vi "KickToPassReceiverTactic.vi"(7 "first call":bool, 8 "error in (no error)":errorcluster, 9 "Robot":refnum<class "Robot.lvclass">, 10 "Game in":refnum<class "Game.lvclass">, 11 "KickToPassReceiverTactic in":refnum<class "KickToPassReceiverTactic.lvclass">) -> (0 "error out":errorcluster, 2 "Robot out":refnum<class "Robot.lvclass">, 3 "KickToPassReceiverTactic out":refnum<class "KickToPassReceiverTactic.lvclass">)   [LabVIEW 2020, in "KickToPassReceiverTactic.lvclass"]
uses:
  KickToPassReceiverTactic.lvclass
  Robot_class/Robot.lvclass
  Game_class/Game.lvclass
  Robot_class/Robot.lvclass/Robot.ctl
  Robot_class/tactics.ctl
  Team_class/OffensivePlay.ctl
  KickToPassReceiverTacticStates.ctl
  Tactic_class/Tactic.lvclass/Tactic.ctl
  Game_class/Game.lvclass/Game.ctl
  Parameters_class/Parameters.lvclass/Parameters.ctl
  Team_class/Team.lvclass/Team.ctl
  Robot_class/roles.ctl
  Object_class/Object.lvclass/Object.ctl
  Skillbook_class/Skillbook.lvclass/Skillbook.ctl
  Events_class/Events.lvclass/Events.ctl
  KickToPassReceiverTactic.lvclass/KickToPassReceiverTactic.ctl
  Robot_class/Read role.vi
  Object_class/Read x.vi
  Object_class/Read y.vi
  Events_class/Read kick.vi
  Events_class/Read touch.vi
  Game_class/Read EventsRef.vi
  Game_class/Read OffensiveTeam.vi
  Team_class/Read OffensivePlay.vi
  Skillbook_class/Read KickToSkill.vi
  Skillbook_class/Read HaltSkill.vi
  Skillbook_class/Read TableReceiverGoToSkill.vi
  Game_class/Read Parameters.lvclass.vi
  Game_class/Read Utilities.lvclass.vi
  Game_class/Read BallRef.vi
  Game_class/Read FieldRef.vi
  Team_class/Read RobotRef.vi
  Parameters_class/Read AttakingOurselves.vi
  Tactic_class/Read Skillbook.vi
  Write States.vi
  Robot_class/Write tactic.vi
  Ally_class/Ally.lvclass
  Ball_class/Ball.lvclass
  Parameters_class/Parameters.lvclass
  Utilities_class/Utilities.lvclass
  Field_class/Field.lvclass
  Skillbook_class/Skillbook.lvclass
  Events_class/Events.lvclass
  KickToSkill_class/KickToSkill.lvclass
  HaltSkill_class/HaltSkill.lvclass
  TableReceiverGoToSkill_class/TableReceiverGoToSkill.lvclass
panel:
  out "x .or. y?":bool
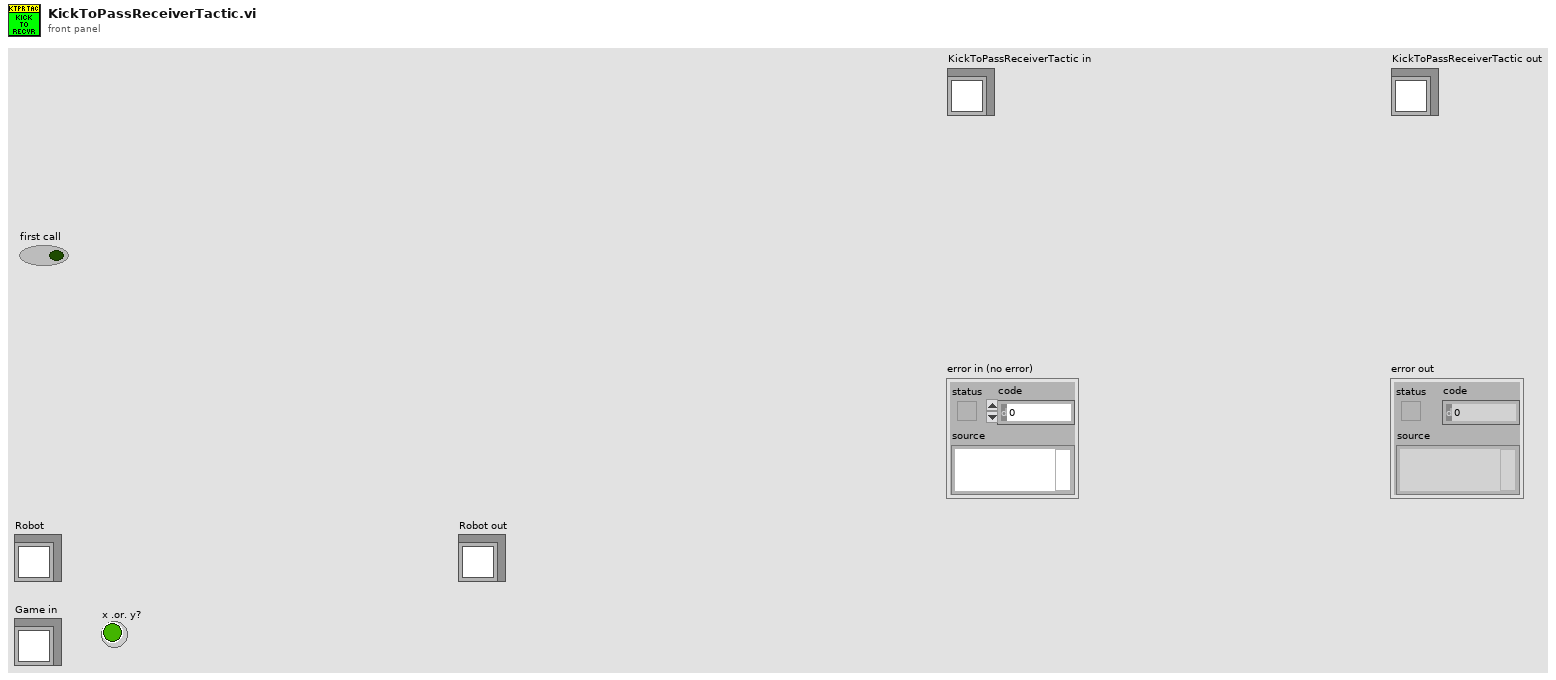
[diagram p1: front panel]
types:
  T1 = typedef "KickToPassReceiverTacticStates.ctl" = enum16{"Halt", "GoToReceiveTable", "KickToPassReceiver", "WaitPass", "Exit"}
  T2 = typedef "OffensivePlay.ctl" = enum16{"KeeperPassToStriker", "PrepareKeeperPass", "ACBPass", "ABCPass", "PrepareTriplePass", "TableWithStriker", "TableWith2ndStrikerPlay", "PrepareDoublePass", "PrepareRollToPass", "SimplePass", "PreparePass", "PassToStriker", "BallOutOfField", "PassTo2ndStriker", "StopOffensive", "Prepare Penalty Enemy", "EnemyPossessionAtEnemyField", "EnemyPossesionAtOurField", "TestPlay", "PreparePenaltyAlly", "KickPenaltyAlly", "PrepareKickoffAlly", "PrepareKickoffEnemy", "IndirectEnemy", "DirectEnemy", "PreparePassInGame1", "NormalGame", "DirectKick", "Pass", "Halt", "Timeout", "PassPlay", "PenaltyEnemy"}
  T3 = typedef "tactics.ctl" = enum16{"ReceivePassInFuturePoint", "Roller", "PrepareRollToPassRollerGoTo", "PrepareRollToPassReceiverGoTo", "WaitRoll", "PositionToRoll", "PenaltyAttacker", "PassObserver", "PenaltyDefense", "TableReceiverTactic", "Test", "DefendGoal", "Marker", "FollowAttacker", "DefendArea", "Shoot", "AttackerAimGoal", "AttackerBallOutOfField", "AttackerBlock", "AttackerStop", "Duelist", "Halt", "ZigZag", "GoTo", "Timeout", "KickToPassReceiver", "PositionToReceivePass", "WaitPass"}
  T4 = typedef "roles.ctl" = enum16{"SecondMarker", "WaitPass", "ABCThirdKicker", "ABCFirstKicker", "ABCSecondKicker", "Tabler", "TableFinalizer", "PrepareRollToPassRoller", "PrepareRollToPassReceiver", "SimplePassRoll", "SimplePassRollReceiver", "PenaltyDefense", "PreparePassReceiver 2", "PreparePassReceiver 1", "PassObserver", "Timeout", "Goto", "ZigZag", "None", "BallOutOfField", "DefenderArea", "Duelist", "AttackerStop", "FollowAttacker", "KeeperRole", "KickPenalty", "AttackerAimGoal", "AttackerBlock", "Marker", "Halt", "Shoot", "PassKicker", "PassReceiver", "TestRole", "PenaltyAttacker"}
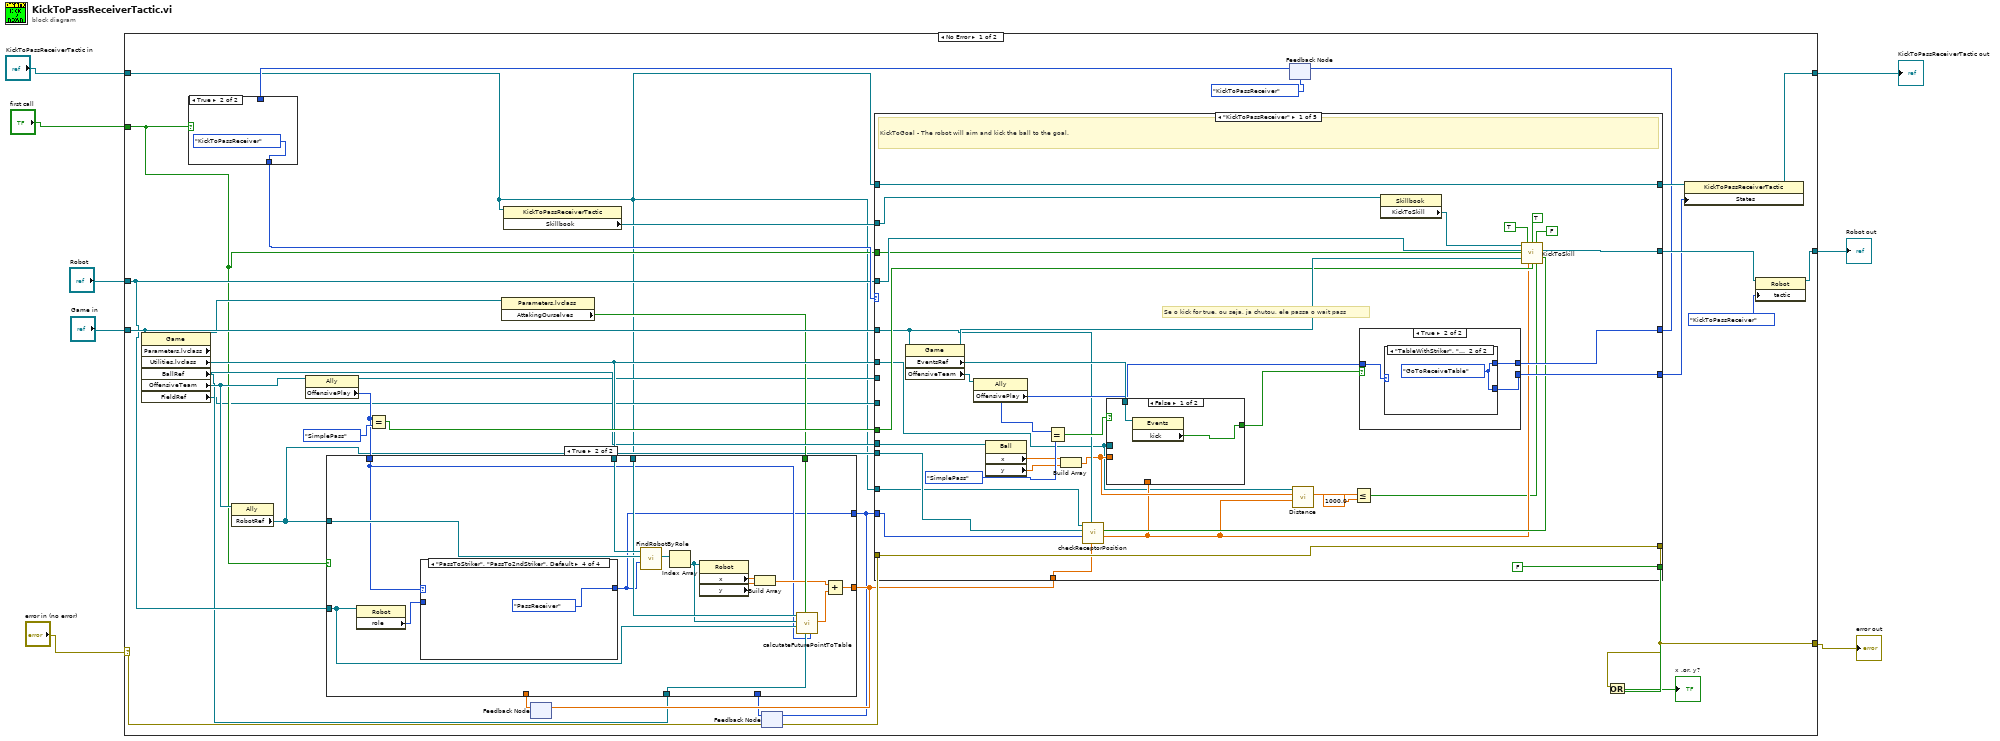
[diagram p0: block diagram]
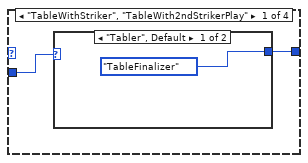
[diagram p3: hidden frame]
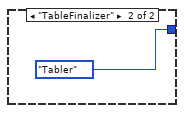
[diagram p4: hidden frame]
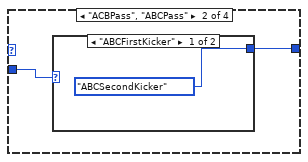
[diagram p5: hidden frame]
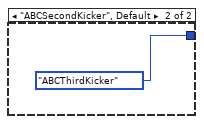
[diagram p6: hidden frame]
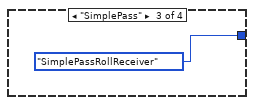
[diagram p7: hidden frame]
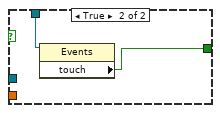
[diagram p9: hidden frame]
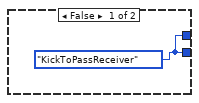
[diagram p10: hidden frame]
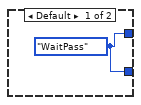
[diagram p11: hidden frame]
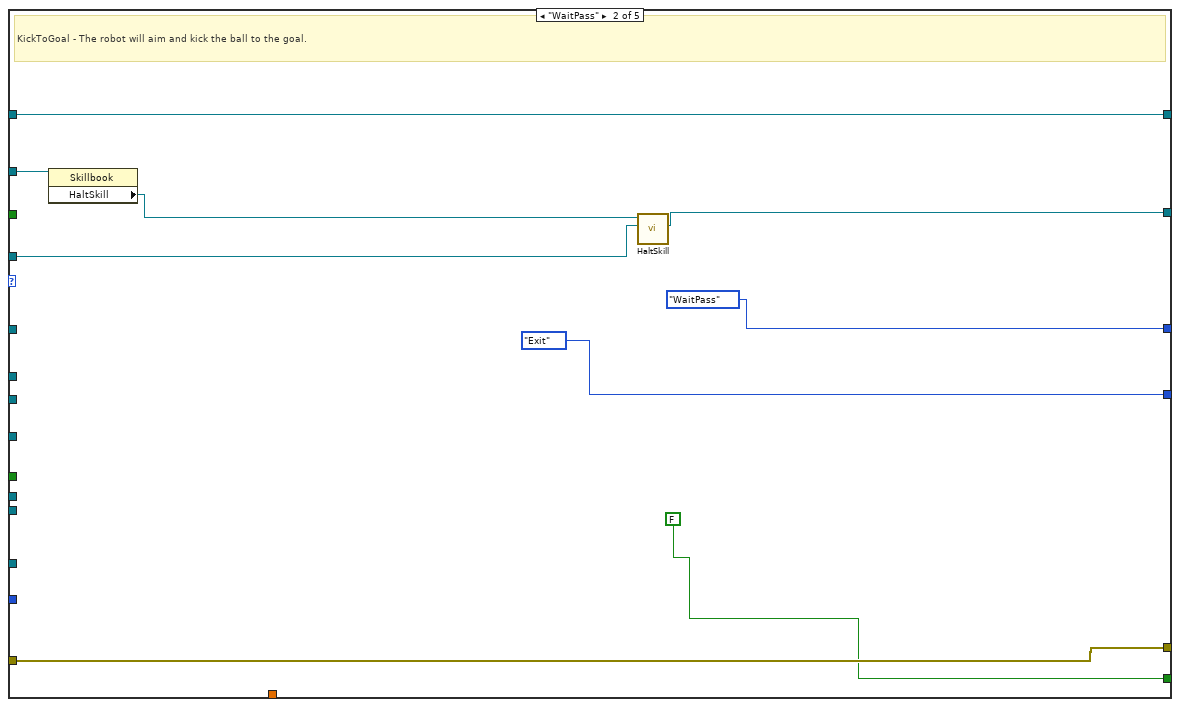
[diagram p12: hidden frame]
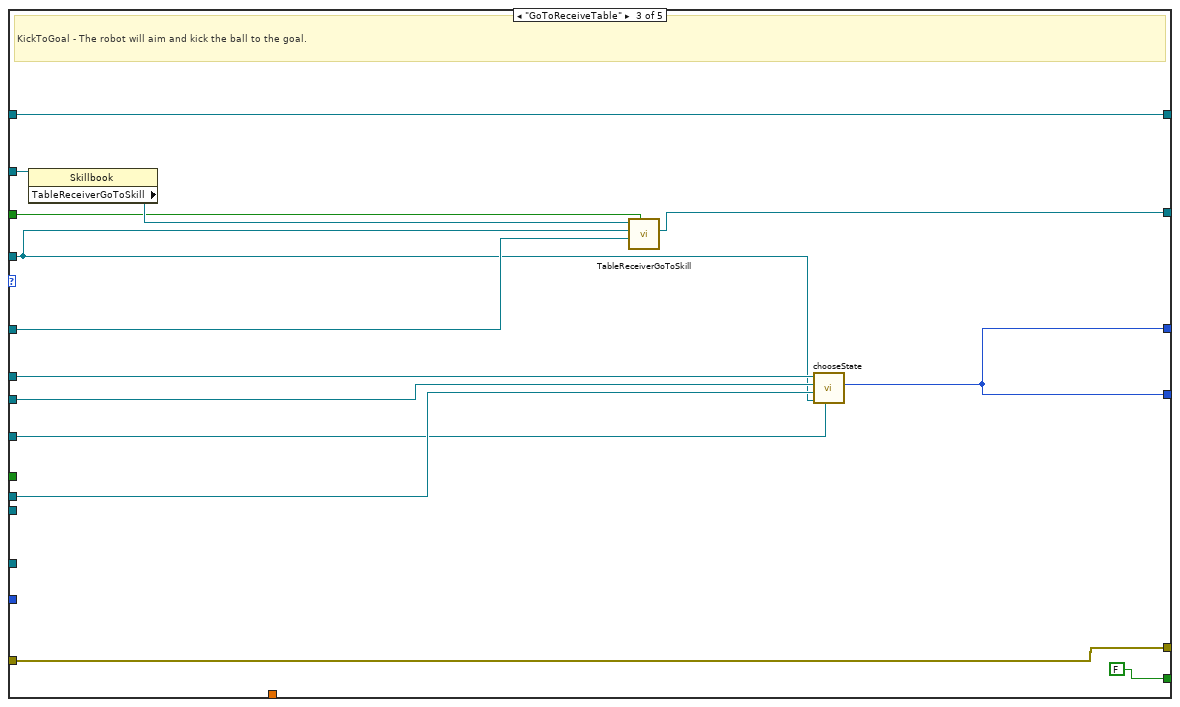
[diagram p13: hidden frame]
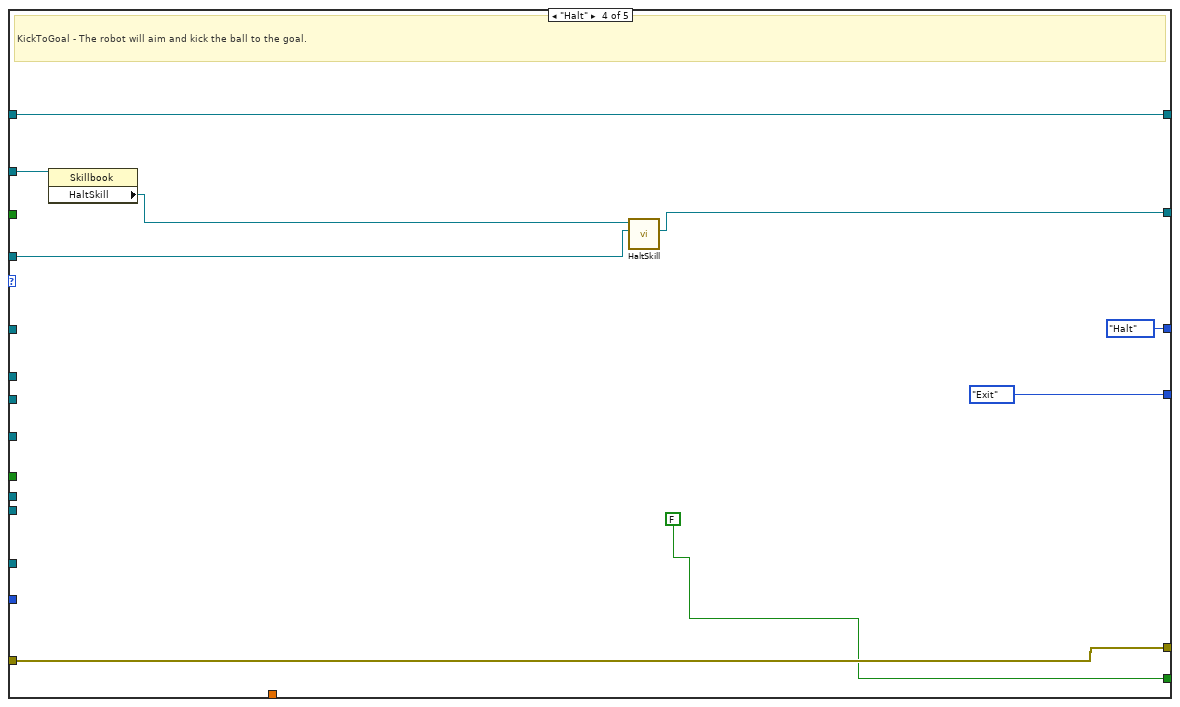
[diagram p14: hidden frame]
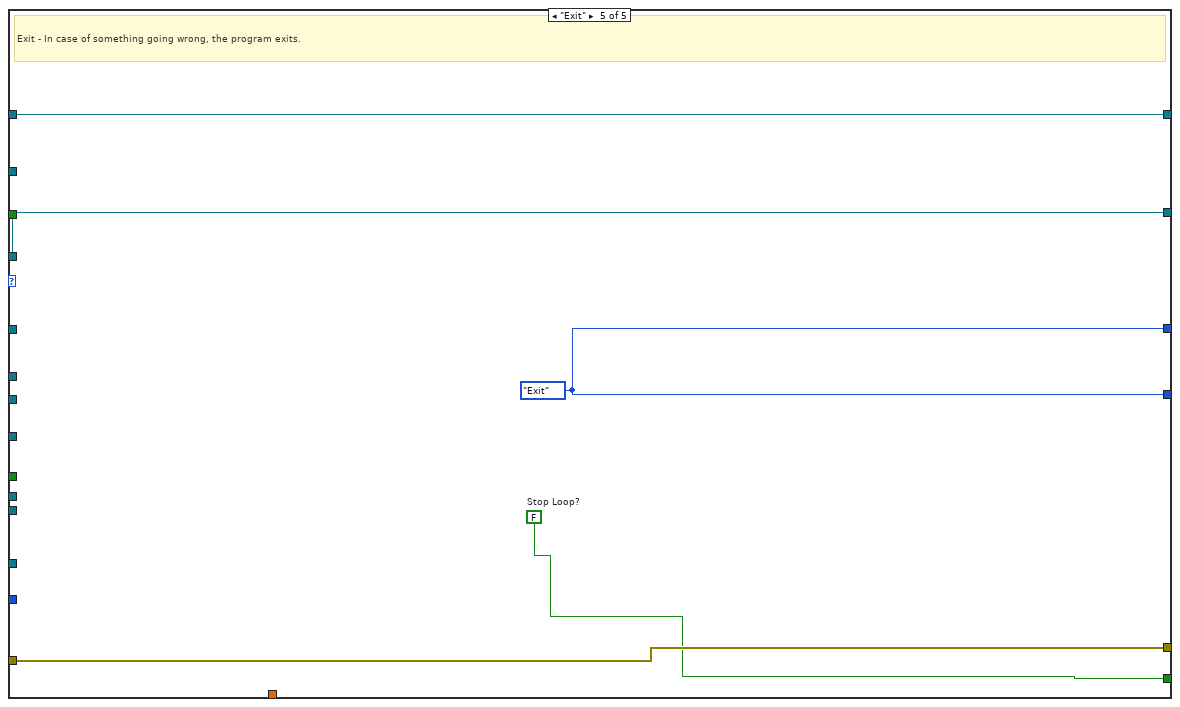
[diagram p15: hidden frame]
diagram:
  n1 = case shown="No Error" "error in (no error)" {
    selector: "error in (no error)" -> [w36 w158]
    tunnel: [w37 w158] -> w2
    tunnel: [w38 w157] -> w3
    tunnel: "KickToPassReceiverTactic in" -> [w9 w157]
    tunnel: "Robot" -> [w23 w156]
    tunnel: "Game in" -> [w35 _]
    tunnel: [w30 w156] -> w6
    tunnel: "first call" -> [w14 _]
    frame No Error {
      n2 = property class="Game"(reference=w35) -> ("Parameters.lvclass"=w20:refnum<class "Parameters.lvclass">, "Utilities.lvclass"=w25:refnum<class "Utilities.lvclass">, "BallRef"=w21:refnum<class "Ball.lvclass">, "OffensiveTeam"=w28:refnum<class "Ally.lvclass">, "FieldRef"=w13:refnum<class "Field.lvclass">)  [unwired: 1 in, 2 out]
      n3 = property class="Ally"(reference=w28) -> ("RobotRef"=w10:refnum<class "Robot.lvclass">[])  [unwired: 1 in, 2 out]
      n4 = property class="Ally"(reference=w28) -> (reference out=w15:refnum<class "Ally.lvclass">, "OffensivePlay"=w24:T2)  [unwired: 1 in, 1 out]
      n5 = Equal?(x=w24, y=OffensivePlay."SimplePass" ("OffensivePlay")) -> (x = y?=w27:bool)
      n6 = property class="Parameters.lvclass"(reference=w20) -> ("AttakingOurselves"=w19:bool)  [unwired: 1 in, 2 out]
      n7 = property class="KickToPassReceiverTactic"(reference=w9) -> ("Skillbook"=w40:refnum<class "Skillbook.lvclass">)  [unwired: 1 in, 2 out]
      n8 = feedback #1() -> (w26:dbl[])  [unwired: 1 in]
      n9 = feedback #2() -> (w11:T4)  [unwired: 1 in]
      n10 = case shown="True" w14 {
        tunnel: w10 -> [_ w60]
        tunnel: w26 -> [w44 _]
        tunnel: w25 -> [_ w59]
        tunnel: w24 -> [_ w46]
        tunnel: w23 -> [_ w48]
        tunnel: [w44 w55] -> w22
        tunnel: w21 -> [_ w47]
        tunnel: w19 -> [_ w52]
        tunnel: w9 -> [_ w51]
        tunnel: [w43 w45] -> w12
        tunnel: w11 -> [w43 _]
        frame False {
        }
        frame True {
          n11 = property class="Robot"(reference=w48) -> ("role"=w54:T4)  [unwired: 1 in, 2 out]
          n12 = case shown="\"PassToStriker\", \"PassTo2ndStriker\", Default" w46 {
            tunnel: [w62 w65 roles."SimplePassRollReceiver" ("role") roles."PassReceiver" ("role")] -> w45
            tunnel: w54 -> [w61 w66 _ _]
            frame "TableWithStriker", "TableWith2ndStrikerPlay" {
              n13 = case shown="\"Tabler\", Default" w61 {
                tunnel: [roles."TableFinalizer" ("role") roles."Tabler" ("role")] -> w62
                frame "Tabler", Default {
                }
                frame "TableFinalizer" {
                }
              }
            }
            frame "ACBPass", "ABCPass" {
              n14 = case shown="\"ABCFirstKicker\"" w66 {
                tunnel: [roles."ABCSecondKicker" ("role") roles."ABCThirdKicker" ("role")] -> w65
                frame "ABCFirstKicker" {
                }
                frame "ABCSecondKicker", Default {
                }
              }
            }
            frame "SimplePass" {
            }
            frame "PassToStriker", "PassTo2ndStriker", Default {
            }
          }
          n15 = call "FindRobotByRole.vi"("role"=w45, "RobotRef"=w60, "Utilities in"=w59) -> ("Robots"=w58:refnum<class "Robot.lvclass">[])  [unwired: 6 in, 2 out]
          n16 = Index Array(array=w58) -> (element=w49:refnum<class "Robot.lvclass">)  [unwired: 1 in]
          n17 = property class="Robot"(reference=w49) -> ("x"=w57:dbl, "y"=w56:dbl)  [unwired: 1 in, 2 out]
          n18 = Build Array(w57, w56) -> (w50:dbl[])
          n19 = call "calcutateFuturePointToTable.vi"("OffensivePlay"=w46, "BallRef"=w47, "AttackingOurselves?"=w52, "Robot that\nmake the pass"=w48, "Robot that will\nreceive the pass"=w49, "KickToPassReceiverTactic in"=w51) -> ("Array to Receiver trajectory"=w53:dbl[])  [unwired: 3 in, 2 out]
          n20 = Add(x=w50, y=w53) -> (x+y=w55:dbl[])
        }
      }
      n21 = feedback-in #1(w22) -> ()
      n22 = feedback-in #2(w12) -> ()
      n23 = feedback #3(KickToPassReceiverTacticStates."KickToPassReceiver" ("States")) -> (w33:T1)
      n24 = case shown="True" w14 {
        tunnel: [w71 KickToPassReceiverTacticStates."KickToPassReceiver" ("States")] -> w34
        tunnel: w33 -> [w71 _]
        frame False {
        }
        frame True {
        }
      }
      n25 = case shown="\"KickToPassReceiver\"" w34 {
        tunnel: [FALSE ("Stop Loop?") FALSE ("Stop Loop?") FALSE ("Stop Loop?") FALSE ("Stop Loop?") w152] -> w42
        tunnel: w36 -> [w107 w125 w137 w145 w155]
        tunnel: [w107 w125 w137 w145 w155] -> w37
        tunnel: w40 -> [w106 w127 w141 w149 _]
        tunnel: w23 -> [w102 w119 w129 w150 w153]
        tunnel: [w104 w121 w139 w147 w153] -> w31
        tunnel: [w105 w126 w138 w146 w154] -> w39
        tunnel: w9 -> [w105 w126 w138 w146 w154]
        tunnel: w35 -> [w80 _ w131 _ _]
        tunnel: [w100 KickToPassReceiverTacticStates."Exit" ("States") w135 KickToPassReceiverTacticStates."Exit" ("States") w151] -> w16
        tunnel: [w99 KickToPassReceiverTacticStates."WaitPass" ("States") w135 KickToPassReceiverTacticStates."Halt" ("States") w151] -> w17
        tunnel: w21 -> [w91 _ w133 _ _]
        tunnel: w25 -> [w76 _ w134 _ _]
        tunnel: w27 -> [w88 _ _ _ _]
        tunnel: w22 -> [w85 _ _ _ _]
        tunnel: w15 -> [_ _ w132 _ _]
        tunnel: w14 -> [w86 _ w130 _ _]
        tunnel: w13 -> [_ _ w128 _ _]
        tunnel: w12 -> [w81 _ _ _ _]
        tunnel: w10 -> [w83 _ _ _ _]
        tunnel: w9 -> [w82 _ _ _ _]
        frame "KickToPassReceiver" {
          # "Se o kick for true, ou seja, ja chutou, ele passa o wait pass"
          # "KickToGoal - The robot will aim and kick the ball to the goal."
          n26 = property class="Game"(reference=w80) -> (reference out=w101:refnum<class "Game.lvclass">, "EventsRef"=w95:refnum<class "Events.lvclass">, "OffensiveTeam"=w93:refnum<class "Ally.lvclass">)  [unwired: 1 in, 1 out]
          n27 = property class="Ally"(reference=w93) -> ("OffensivePlay"=w87:T2)  [unwired: 1 in, 2 out]
          n28 = property class="Ball"(reference=w91) -> ("x"=w90:dbl, "y"=w89:dbl)  [unwired: 1 in, 2 out]
          n29 = Equal?(x=w87, y=OffensivePlay."SimplePass" ("OffensivePlay")) -> (x = y?=w96:bool)
          n30 = Build Array(w90, w89) -> (w78:dbl[])
          n31 = call "checkReceptorPosition.vi"("target"=w85, "Game"=w80, "role"=w81, "OffensiveRobots"=w83, "KickToPassReceiverTactic in"=w82) -> ("finalTarget"=w77:dbl[], "calculateForce"=w84:bool)  [unwired: 3 in, 2 out]
          n32 = case shown="False" w96 {
            tunnel: w95 -> [w110 w112]
            tunnel: [w109 w111] -> w94
            tunnel: w77 -> [_ _]
            tunnel: w78 -> [_ _]
            tunnel: w76 -> [_ _]
            frame False {
              n33 = property class="Events"(reference=w110) -> ("kick"=w109:bool)  [unwired: 1 in, 2 out]
            }
            frame True {
              n34 = property class="Events"(reference=w112) -> ("touch"=w111:bool)  [unwired: 1 in, 2 out]
            }
          }
          n35 = call-dynamic "Distance.vi"("P1"=w77, "P2"=w78, "Utilities in"=w76) -> ("Distance"=w75:dbl)  [unwired: 6 in, 2 out]
          n36 = Less Or Equal?(x=w75, y=1000.0) -> (x <= y?=w73:bool)
          n37 = case shown="True" w94 {
            tunnel: [w113 w116] -> w100
            tunnel: [w113 w115] -> w99
            tunnel: w87 -> [_ w114]
            frame False {
              w113 = KickToPassReceiverTacticStates."KickToPassReceiver" ("States")
            }
            frame True {
              n38 = case shown="\"TableWithStriker\", \"TableWith2ndStrikerPlay\"" w114 {
                tunnel: [w117 w118] -> w116
                tunnel: [w117 w118] -> w115
                frame Default {
                  w117 = KickToPassReceiverTacticStates."WaitPass" ("States")
                }
                frame "TableWithStriker", "TableWith2ndStrikerPlay" {
                  w118 = KickToPassReceiverTacticStates."GoToReceiveTable" ("States")
                }
              }
            }
          }
          n39 = property class="Skillbook"(reference=w106) -> ("KickToSkill"=w103:refnum<class "KickToSkill.lvclass">)  [unwired: 1 in, 2 out]
          n40 = call "KickToSkill.vi"("KickToSkill in"=w103, "use criteria?"=TRUE, "chipKick ?"=TRUE, "fixTarget"=FALSE, "Robot"=w102, "firstCall?"=w86, "Game"=w101, "calculate force?"=w84, "Target"=w77, "KickForce 0?"=w88, "ForceInGame"=w73) -> ("Robot out"=w104:refnum<class "Robot.lvclass">)  [unwired: 2 in, 2 out]
        }
        frame "WaitPass" {
          # "KickToGoal - The robot will aim and kick the ball to the goal."
          n41 = property class="Skillbook"(reference=w127) -> ("HaltSkill"=w120:refnum<class "HaltSkill.lvclass">)  [unwired: 1 in, 2 out]
          n42 = call-dynamic "HaltSkill.vi"("Robot"=w119, "HaltSkill in"=w120) -> ("Robot out"=w121:refnum<class "Robot.lvclass">)  [unwired: 7 in, 2 out]
        }
        frame "GoToReceiveTable" {
          # "KickToGoal - The robot will aim and kick the ball to the goal."
          n43 = property class="Skillbook"(reference=w141) -> ("TableReceiverGoToSkill"=w140:refnum<class "TableReceiverGoToSkill.lvclass">)  [unwired: 1 in, 2 out]
          n44 = call "TableReceiverGoToSkill.vi"("Firstcall?"=w130, "Game"=w131, "Robot in"=w129, "TableReceiverGoToSkill in"=w140) -> ("Robot out"=w139:refnum<class "Robot.lvclass">)  [unwired: 5 in, 2 out]
          n45 = call "chooseState.vi"("FieldRef"=w128, "Robot"=w129, "BallRef"=w133, "OffensiveTeam"=w132, "Utilities in"=w134) -> ("state"=w135:T1)  [unwired: 6 in]
        }
        frame "Halt" {
          # "KickToGoal - The robot will aim and kick the ball to the goal."
          n46 = property class="Skillbook"(reference=w149) -> ("HaltSkill"=w148:refnum<class "HaltSkill.lvclass">)  [unwired: 1 in, 2 out]
          n47 = call-dynamic "HaltSkill.vi"("Robot"=w150, "HaltSkill in"=w148) -> ("Robot out"=w147:refnum<class "Robot.lvclass">)  [unwired: 7 in, 2 out]
        }
        frame "Exit" {
          w151 = KickToPassReceiverTacticStates."Exit" ("States")
          w152 = FALSE  # Stop Loop?
          # "Exit - In case of something going wrong, the program exits."
        }
      }
      n48 = feedback-in #3(w17) -> ()
      n49 = Or(x=w37, y=w42) -> (x .or. y?=→"x .or. y?":bool)
      n50 = property class="KickToPassReceiverTactic"(reference=w39, "States"=w16) -> (reference out=w38:refnum<class "KickToPassReceiverTactic.lvclass">)  [unwired: 1 in, 1 out]
      n51 = property class="Robot"(reference=w31, "tactic"=tactics."KickToPassReceiver") -> (reference out=w30:refnum<class "Robot.lvclass">)  [unwired: 1 in, 1 out]
    }
    frame Error {
    }
  }
  "error out" <- w2
  "KickToPassReceiverTactic out" <- w3
  "Robot out" <- w6
